vi "get precedence.vi"(3 "operator":string) -> (1 "Precedence":i32)   [LabVIEW 2020]
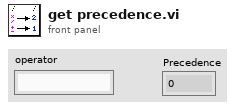
[diagram p1: front panel]
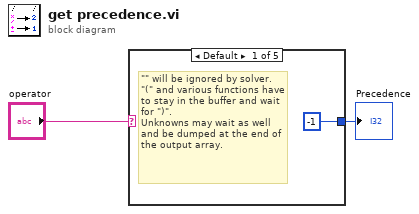
[diagram p0: block diagram]
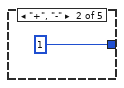
[diagram p2: hidden frame]
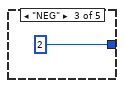
[diagram p3: hidden frame]
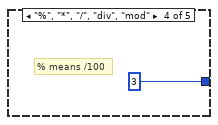
[diagram p4: hidden frame]
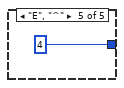
[diagram p5: hidden frame]
diagram:
  n1 = case shown="Default" "operator" {
    tunnel: [-1 1 2 3 4] -> w1
    frame Default {
      # "\"\" will be ignored by solver.\n\"(\" and various functions have to stay in the buffer and wait for \")\". \nUnknowns may wait as well and be dumped at the end of the output array."
    }
    frame "+", "-" {
    }
    frame "NEG" {
    }
    frame "%", "*", "/", "div", "mod" {
      # "% means /100"
    }
    frame "E", "^" {
    }
  }
  "Precedence" <- w1
